vi "Configure.vi"(4 "error in":errorcluster, 5 "timeout":i32=5000, 6 "source":string, 7 "ref in":refnum<k7>) -> (0 "error out":errorcluster, 3 "ref out":refnum<k7>)   [LabVIEW 2010]
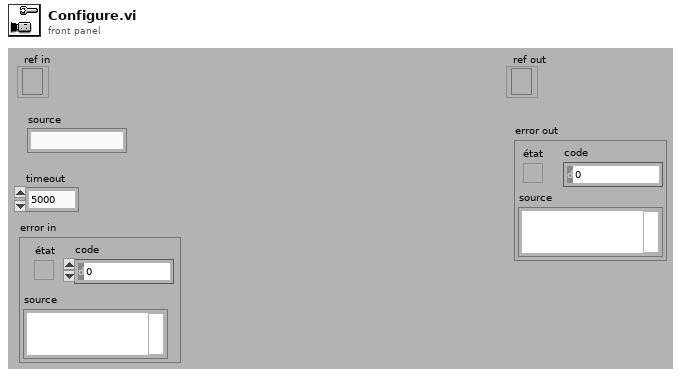
[diagram p1: front panel]
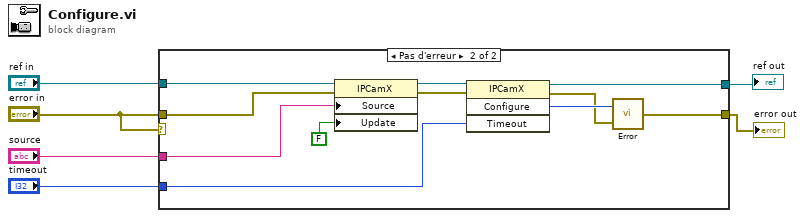
[diagram p0: block diagram]
diagram:
  n1 = case shown="Pas d'erreur" "error in" {
    tunnel: "source" -> [_ w14]
    tunnel: [w7 w9] -> w5
    tunnel: [w8 w12] -> w4
    tunnel: "timeout" -> [_ w13]
    tunnel: "error in" -> [w7 w15]
    tunnel: "ref in" -> [w8 w16]
    frame Error {
    }
    frame No Error {
      n2 = property class="IPCamX"(reference=w16, error in=w15, "Source"=w14, "Update"=FALSE) -> (reference out=w19:refnum<k7>, error out=w18:errorcluster)
      n3 = invoke class="IPCamX" method="Configure"(reference=w19, error in=w18, "Timeout"=w13) -> (reference out=w12:refnum<k7>, error out=w10:errorcluster, "Configure"=w11:i32)  [unwired: 1 in, 1 out]
      n4 = call "Error.vi"("error in"=w10, "code"=w11) -> ("error out"=w9:errorcluster)
    }
  }
  "error out" <- w5
  "ref out" <- w4
